vi "Set Waveform Display Intensity.vi"(8 "error in (no error)":errorcluster, 10 "Intensity (1-100)":i8=1 min=1 max=100 step=1, 11 "PXIe5105 in":refnum<class "PXIe5105.lvclass">) -> (0 "error out":errorcluster, 3 "PXIe5105 out":refnum<class "PXIe5105.lvclass">)   [LabVIEW 2018, in "PXIe5105.lvlib" / "PXIe5105.lvclass"]
doc: "This Override is used to change the display intensity level for the oscilloscope waveforms."
uses:
  PXIe5105.lvclass
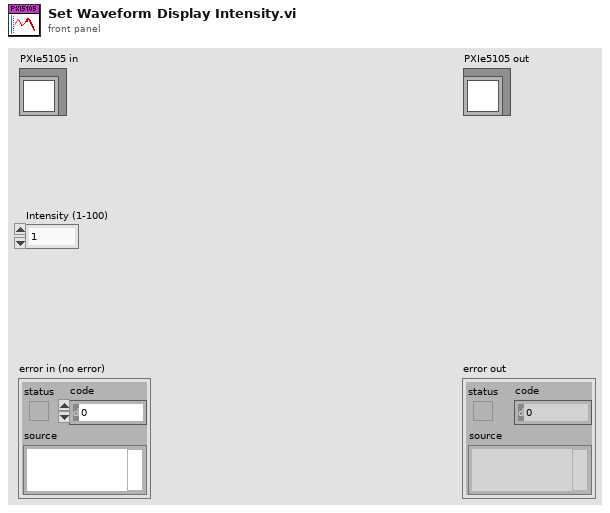
[diagram p1: front panel]
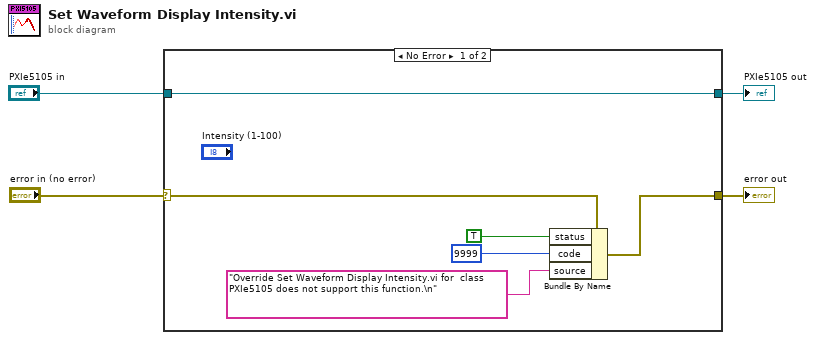
[diagram p0: block diagram]
diagram:
  n1 = case shown="No Error" "error in (no error)" {
    selector: "error in (no error)" -> [w7 w12]
    tunnel: [w5 w12] -> w3
    tunnel: [w6 w11] -> w2
    tunnel: "PXIe5105 in" -> [w6 w11]
    frame No Error {
      n2 = Bundle By Name(cluster=w7, "status"=TRUE, "code"=9999, "source"="Override Set Waveform Display Intensity.vi for  class PXIe5105 does not support this function.\n") -> (w5:errorcluster)
    }
    frame Error {
    }
  }
  "error out" <- w3
  "PXIe5105 out" <- w2
